vi "UnitTest.vi"() -> ()   [LabVIEW 2018]
uses:
  Libraries/Example/Do Something Else and Wait (Reply Payload)--cluster.ctl
  ExampleAPI.lvclass
  Libraries/Example/Example.lvlib
panel:
  out "Close Session":u32
  out "Do Something Else and Wait for Reply":u32
  out "Open Session":u32
  in  "Iterations":i32=200
  out "N Iteration of Do Something":u32
  out "Reply Payload":T1
  out "timed out?":bool
  in  "X":dbl
  in  "wait for reply (T)":bool=TRUE
  in  "Do Something Message":string
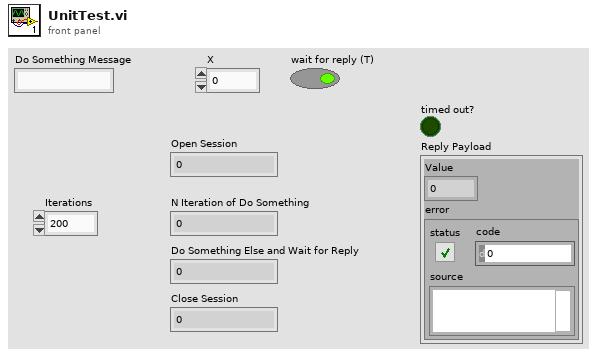
[diagram p1: front panel]
types:
  T1 = typedef "Example.lvlib/Do Something Else and Wait (Reply Payload)--cluster.ctl" = cluster{"Value":dbl, "error":errorcluster}
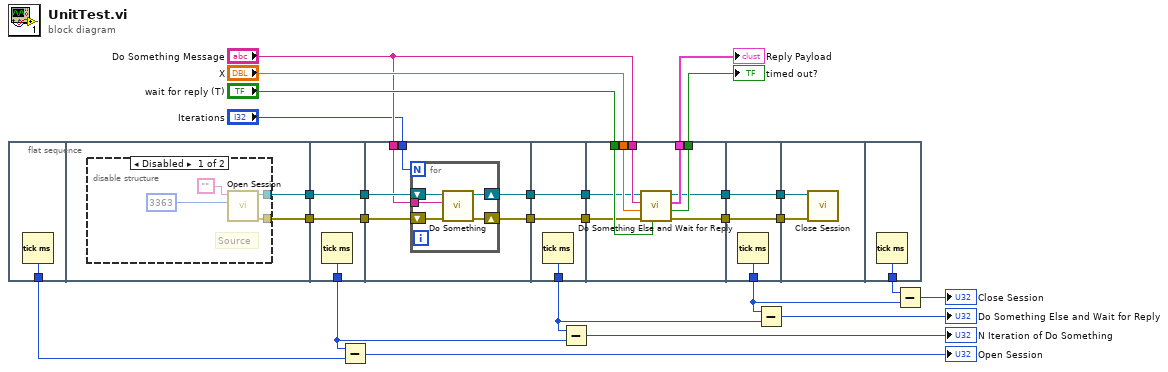
[diagram p0: block diagram]
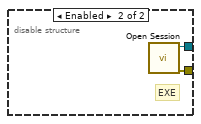
[diagram p2: hidden frame]
diagram:
  n1 = flat-sequence {
    tunnel: [w28] -> w19
    tunnel: [w30] -> w22
    tunnel: [w29] -> w2
    tunnel: [w39] -> w25
    tunnel: [w38] -> w24
    tunnel: [w37] -> w20
    tunnel: w22 -> [w38]
    tunnel: w2 -> [w39]
    tunnel: [w43] -> w27
    tunnel: [w42] -> w26
    tunnel: w25 -> [w45]
    tunnel: w24 -> [w44]
    tunnel: "Iterations" -> [w41]
    tunnel: "Do Something Message" -> [w40]
    tunnel: w27 -> [w53]
    tunnel: w26 -> [w52]
    tunnel: [w53] -> w18
    tunnel: [w52] -> w17
    tunnel: [w51] -> w4
    tunnel: w18 -> [w58]
    tunnel: w17 -> [w61]
    tunnel: "wait for reply (T)" -> [w62]
    tunnel: "X" -> [w60]
    tunnel: "Do Something Message" -> [w59]
    tunnel: [w56] -> w13
    tunnel: [w55] -> w12
    tunnel: [w57] -> w11
    tunnel: [w54] -> w10
    tunnel: w11 -> [w65]
    tunnel: w10 -> [w64]
    tunnel: [w63] -> w3
    tunnel: [w65] -> w8
    tunnel: [w64] -> w7
    tunnel: w8 -> [w66]
    tunnel: w7 -> [w67]
    tunnel: [w68] -> w5
    frame #0 {
      n2 = Tick Count (ms)() -> (millisecond timer value=w28:u32)
    }
    frame #1 {
      n3 = disable-structure shown="Disabled" {
        disable-tunnel: [w34 w36] -> w30
        disable-tunnel: [w33 w35] -> w29
        frame Disabled {
          # "Source"
          n4 = call "Open Session.vi"("port number or service name (3364)"=u16 3363, "machine name (\"\":  local reference)"="" ("machine name (\"\":  local reference)")) -> ("error out"=w34:errorcluster, "ExampleAPI out"=w33:refnum<class "ExampleAPI.lvclass">)  [unwired: 8 in]
        }
        frame Enabled {
          # "EXE"
          n5 = call "Open Session.vi"() -> ("error out"=w36:errorcluster, "ExampleAPI out"=w35:refnum<class "ExampleAPI.lvclass">)  [unwired: 10 in]
        }
      }
    }
    frame #2 {
      n6 = Tick Count (ms)() -> (millisecond timer value=w37:u32)
    }
    frame #3 {
      n7 = for {
        N: w41 -> [_]
        tunnel: w40 -> [w46]
        shift-right: [w48] -> w43
        shift-left: w45 -> [w50]
        shift-right: [w47] -> w42
        shift-left: w44 -> [w49]
        n8 = call "Do Something.vi"("error in (no error)"=w49, "Do Something Message"=w46, "TemplateAPI in"=w50) -> ("error out"=w47:errorcluster, "TemplateAPI out"=w48:refnum<class "ExampleAPI.lvclass">)  [unwired: 7 in]
      }
    }
    frame #4 {
      n9 = Tick Count (ms)() -> (millisecond timer value=w51:u32)
    }
    frame #5 {
      n10 = call "Do Something Else and Wait for Reply.vi"("wait for reply (T)"=w62, "error in (no error)"=w61, "X"=w60, "Do Something Message"=w59, "TemplateAPI in"=w58) -> ("error out"=w57:errorcluster, "timed out?"=w56:bool, "Reply Payload"=w55:T1, "TemplateAPI out"=w54:refnum<class "ExampleAPI.lvclass">)  [unwired: 3 in]
    }
    frame #6 {
      n11 = Tick Count (ms)() -> (millisecond timer value=w63:u32)
    }
    frame #7 {
      n12 = call "Close Session.vi"("error in (no error)"=w66, "ExampleAPI.lvclass"=w67) -> ()  [unwired: 9 in, 1 out]
    }
    frame #8 {
      n13 = Tick Count (ms)() -> (millisecond timer value=w68:u32)
    }
  }
  n14 = Subtract(x=w20, y=w19) -> (x-y=→"Open Session":u32)
  n15 = Subtract(x=w4, y=w20) -> (x-y=→"N Iteration of Do Something":u32)
  n16 = Subtract(x=w3, y=w4) -> (x-y=→"Do Something Else and Wait for Reply":u32)
  n17 = Subtract(x=w5, y=w3) -> (x-y=→"Close Session":u32)
  "timed out?" <- w13
  "Reply Payload" <- w12
